vi "Flatten Value.vi"(8 "Error In":errorcluster, 11 "Bool Array In":refnum<class "1D Bool.lvclass">) -> (0 "Error Out":errorcluster, 1 "Value":string, 3 "Bool Array Out":refnum<class "1D Bool.lvclass">)   [LabVIEW 2017, in "Tree API.lvlib" / "1D Bool.lvclass"]
uses:
  1D Bool.lvclass
  Tree Manager/Tree.lvclass
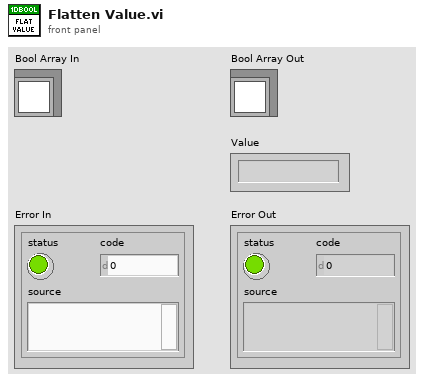
[diagram p1: front panel]
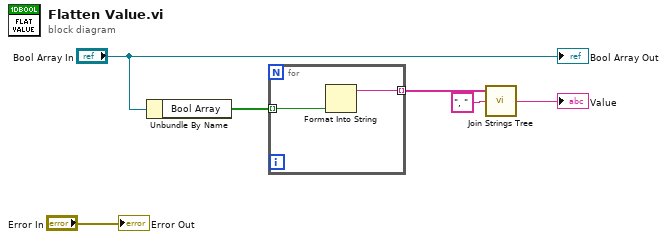
[diagram p0: block diagram]
diagram:
  n1 = Unbundle By Name("Bool Array In") -> ("Bool Array"=w5:bool[])
  n2 = for {
    tunnel: w5 -> [w8] mode=indexing
    tunnel: [w7] -> w3 mode=indexing
    n3 = Format Into String(w8) -> (resulting string=w7:string)  [unwired: 3 in, 1 out]
  }
  n4 = call "Join Strings Tree.vi"("Separator (,)"=", ", "Strings In"=w3) -> ("String"=→"Value":string)  [unwired: 1 in]
  "Bool Array Out" <- "Bool Array In"
  "Error Out" <- "Error In"
